vi "Set DataSend.vi"(8 "error in (no error)":errorcluster caption="entrée d'erreur (pas d'erreur)", 10 "DataSend":T1, 11 "Client TCP_IP P2110 en entrée":refnum<class "Client TCP_IP P2110.lvclass">) -> (0 "error out":errorcluster caption="sortie d'erreur", 3 "Client TCP_IP P2110 en sortie":refnum<class "Client TCP_IP P2110.lvclass">)   [LabVIEW 2020, in "Library Instrument & Equipement.lvlib" / "Library TCP IP.lvlib" / "Client TCP_IP P2110.lvclass"]
uses:
  Client TCP_IP P2110.lvclass
  C:/Users/ngarcin/OneDrive - Altyor/Standard TB/Class/TCP IP/Client TCP_IP (Default)/Dossier Client TCP_IP (Default)/Client TCP_IP (Default).lvclass
  Client TCP_IP P2110.lvclass/Client TCP_IP P2110.ctl
  JSON API/Variant JSON/Variant to JSON.vi
  JSON API/JSON Value/Get Item by name array.vi
  JSON API/JSON Value/JSON Value.lvclass
  JSON API/Get Polymorphic/JSON GetSet.lvlib
  JSON API/Variant JSON/Variant JSON.lvlib
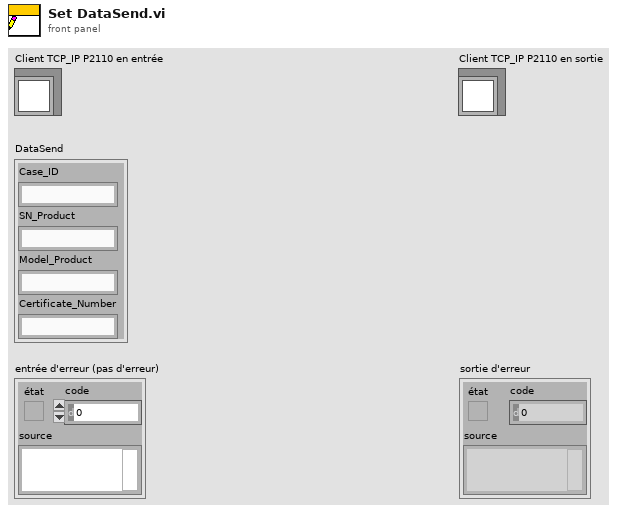
[diagram p1: front panel]
types:
  T1 = cluster{"Case_ID":string, "SN_Product":string, "Model_Product":string, "Certificate_Number":string}
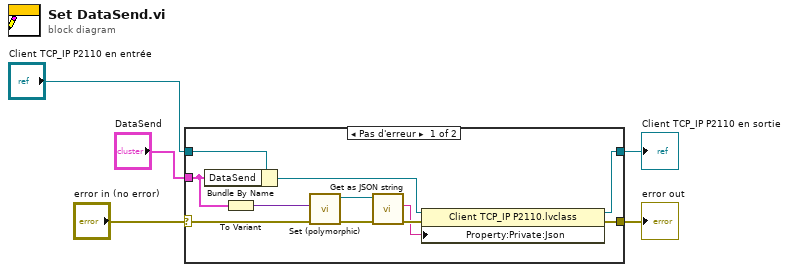
[diagram p0: block diagram]
diagram:
  n1 = case shown="Pas d'erreur" "error in (no error)" {
    selector: "error in (no error)" -> [w7 w17]
    tunnel: [w6 w17] -> w4
    tunnel: [w8 w18] -> w2
    tunnel: "Client TCP_IP P2110 en entrée" -> [w16 w18]
    tunnel: "DataSend" -> [w10 _]
    frame No Error {
      n2 = Bundle By Name(cluster=w16, "DataSend"=w10) -> (w9:refnum<class "Client TCP_IP P2110.lvclass">)
      n3 = To Variant(anything=w10) -> (Variant=w15:variant)
      n4 = call-poly "Set (polymorphic).vi"("error in (no error)"=w7, "Variant"=w15) -> ("error out"=w13:errorcluster, "JSON Value out"=w14:refnum<class "JSON Value.lvclass">)  [unwired: 8 in]
      n5 = call "Get as JSON string.vi"("error in (no error)"=w13, "JSON Value in"=w14) -> ("error out"=w12:errorcluster, "<JSON>"=w11:string)  [unwired: 8 in]
      n6 = property class="Client TCP_IP P2110.lvclass"(reference=w9, error in=w12, "Property:Private:Json"=w11) -> (reference out=w8:refnum<class "Client TCP_IP P2110.lvclass">, error out=w6:errorcluster)
    }
    frame Error {
    }
  }
  "error out" <- w4
  "Client TCP_IP P2110 en sortie" <- w2
